vi "Write Button Height.vi"(8 "error in (no error)":errorcluster, 10 "Button Height":i32, 11 "Toolbar Control in":refnum<class "Toolbar Control.lvclass">) -> (0 "error out":errorcluster, 3 "Toolbar Control out":refnum<class "Toolbar Control.lvclass">)   [LabVIEW 2011, in "Toolbar Control.lvclass"]
doc: "-------------\nDeveloped by Brian Hoover (hooovahh)"
uses:
  Toolbar Control.lvclass
  Toolbar Control.lvclass/Toolbar Control.ctl
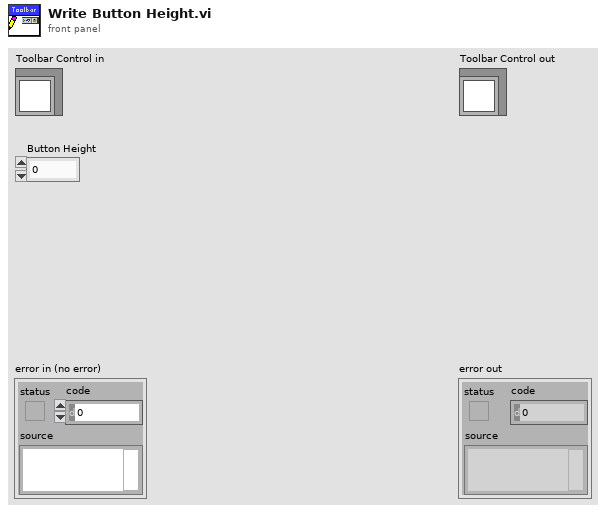
[diagram p1: front panel]
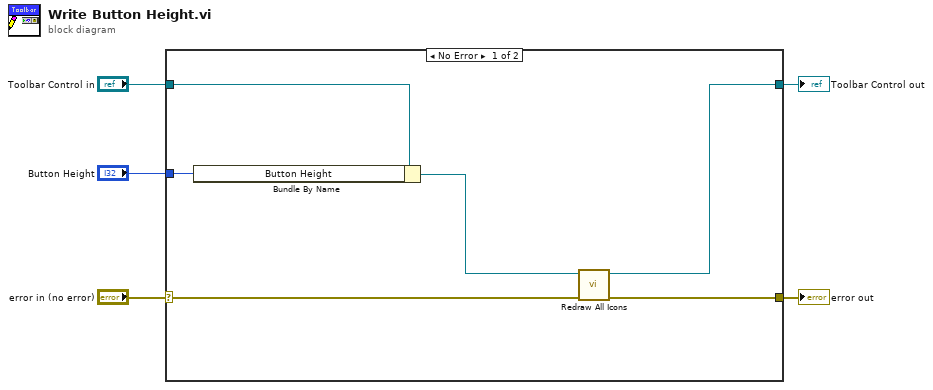
[diagram p0: block diagram]
diagram:
  n1 = case shown="No Error" "error in (no error)" {
    selector: "error in (no error)" -> [w8 w12]
    tunnel: [w7 w12] -> w4
    tunnel: [w6 w13] -> w2
    tunnel: "Toolbar Control in" -> [w10 w13]
    tunnel: "Button Height" -> [w11 _]
    frame No Error {
      n2 = Bundle By Name(cluster=w10, "Button Height"=w11) -> (w9:refnum<class "Toolbar Control.lvclass">)
      n3 = call "Redraw All Icons.vi"("error in (no error)"=w8, "Toolbar Control in"=w9) -> ("error out"=w7:errorcluster, "Toolbar Control out"=w6:refnum<class "Toolbar Control.lvclass">)  [unwired: 7 in, 1 out]
    }
    frame Error {
    }
  }
  "error out" <- w4
  "Toolbar Control out" <- w2
